vi "ps_queue.vi"(8 "error in (no error)":errorcluster) -> (0 "error out":errorcluster)   [LabVIEW 2013]
uses:
  main_machine/type_defs/mm_states.ctl
panel:
  out "MM_STATE":refnum<queue>
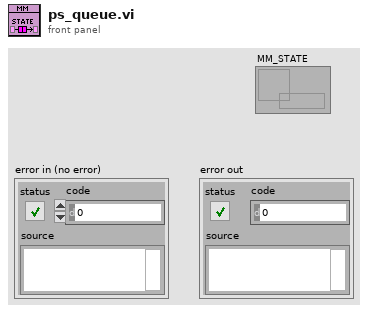
[diagram p1: front panel]
types:
  T1 = typedef "mm_states.ctl" = enum16{"STARTUP", "WAIT FOR COMMAND", "INITIALIZE INSTRUMENT", "FIND FCS FILE ", "START EXPERIMENT", "WAIT TO SAMPLE ", "DILUTE", "TAKE SAMPLE ", "EXIT"}
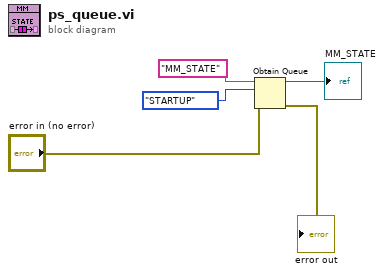
[diagram p0: block diagram]
diagram:
  n1 = Obtain Queue(name (unnamed)="MM_STATE", element data type=mm_states."STARTUP" ("Enum"), error in (no error)="error in (no error)") -> (queue out=→"MM_STATE":refnum<queue>, error out=→"error out":errorcluster)  [unwired: 2 in, 1 out]
